vi "参数设置对画框.vi"(8 "时间等比采样":u16=10, 9 "单次采样量":u16=500, 10 "采样方式":enum16{"单采", "双重"}(ring), 11 "留样模式":T1(ring)=enum."外控留样") -> ()   [LabVIEW 2016, in "德润DR803L超标留样.lvlib"]
uses:
  <vilib>/Utility/config.llb/NI_LVConfig.lvlib
panel:
  in  "关闭":bool
  in  "打开串口":bool
  in  "释放串口":bool
  in  "超标浓度配置":bool
  # "只在停止时切换有效"
  # "只在待机时切换有效"
  # "默认：500ml（5-1000）ml （只在停止时写有效）"
  # "默认：10min（2-9999）min （只在停止时写有效）"
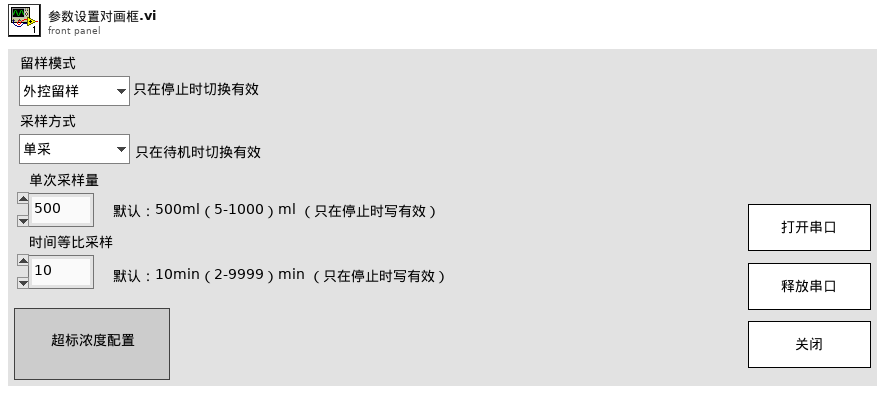
[diagram p1: front panel]
types:
  T1 = enum16{"无", "定时留样", "时间等比例", "超标留样", "同步留样", "外控留样"}
  T2 = enum16{"open", "read", "write", "write single", "close"}
  T3 = cluster{"氨氮超标浓度":dbl, "总磷超标浓度":dbl, "总氮超标浓度":dbl, "CODMn超标浓度":dbl, "CODCr超标浓度":dbl, "PH超标浓度":dbl, "DO超标浓度":dbl, "SPCOND超标浓度":dbl, "浊度超标浓度":dbl, "叶绿素a超标浓度":dbl, "蓝绿藻超标浓度":dbl, "藻密度超标浓度":dbl, "ORP超标浓度":dbl, "COD超标浓度":dbl}
  T4 = typedef "NI_LVConfig.lvlib/Config Data RefNum.ctl" = refnum<k1>
  T5 = cluster{"确定":bool, "氨氮超标浓度":dbl, "总磷超标浓度":dbl, "总氮超标浓度":dbl, "CODMn超标浓度":dbl, "CODCr超标浓度":dbl, "PH超标浓度":dbl, "DO超标浓度":dbl, "SPCOND超标浓度":dbl, "浊度超标浓度":dbl, "叶绿素a超标浓度":dbl, "蓝绿藻超标浓度":dbl, "藻密度超标浓度":dbl, "ORP超标浓度":dbl, "COD超标浓度":dbl}
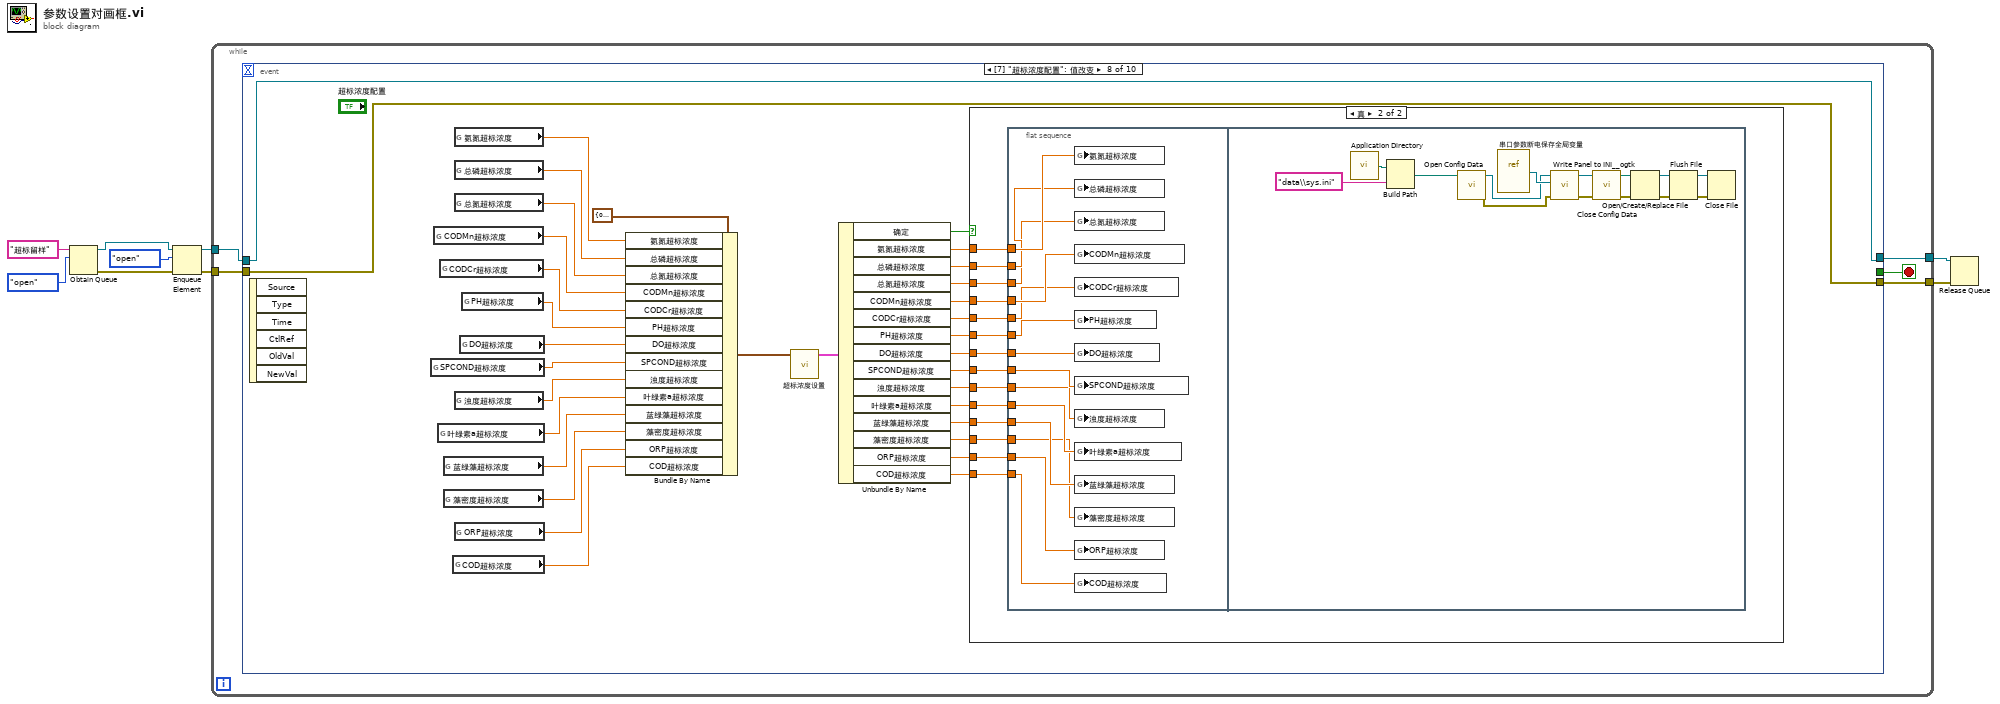
[diagram p0: block diagram]
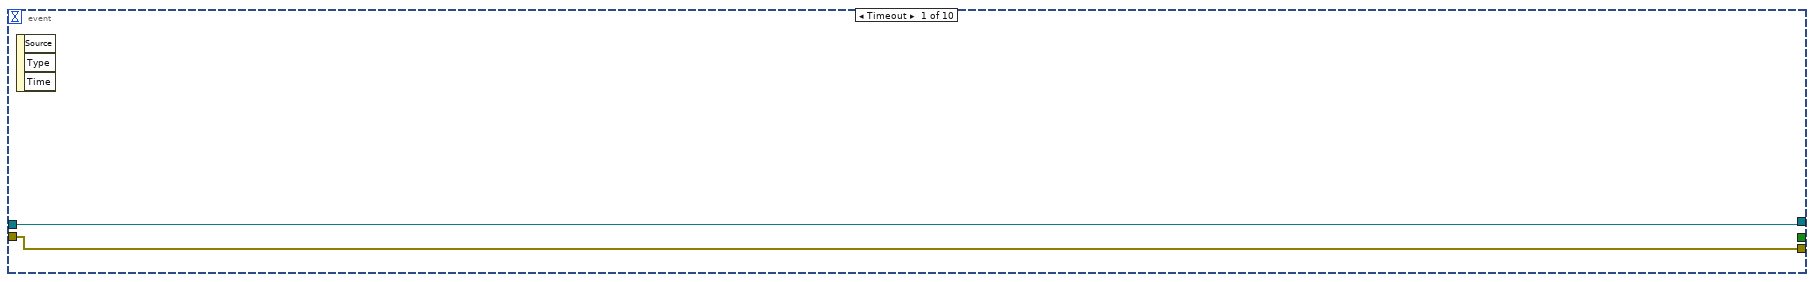
[diagram p2: hidden frame]
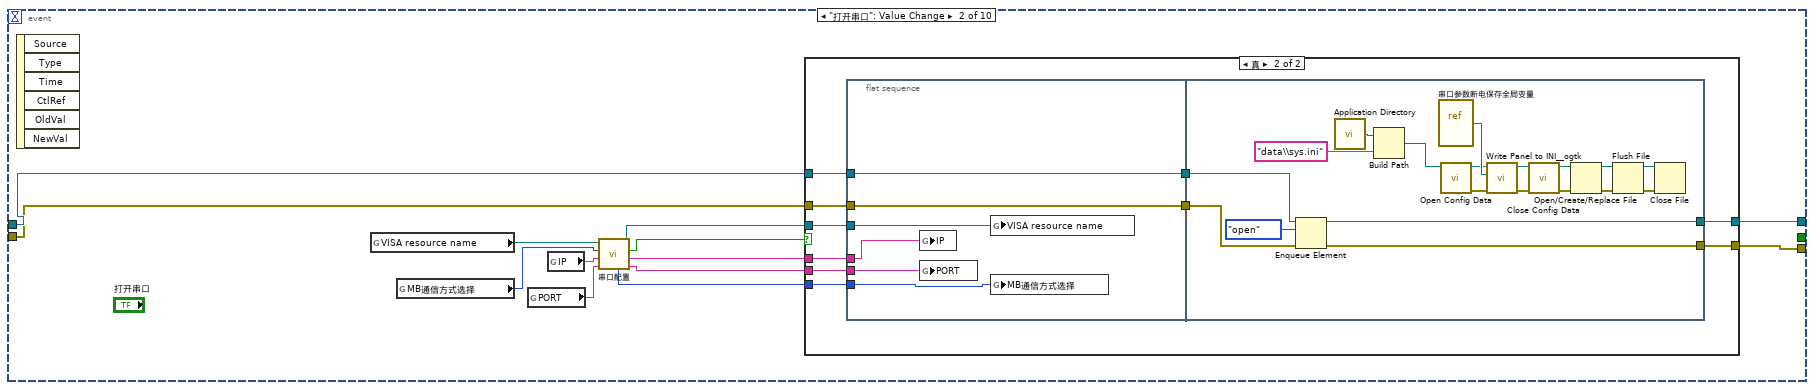
[diagram p3: hidden frame]
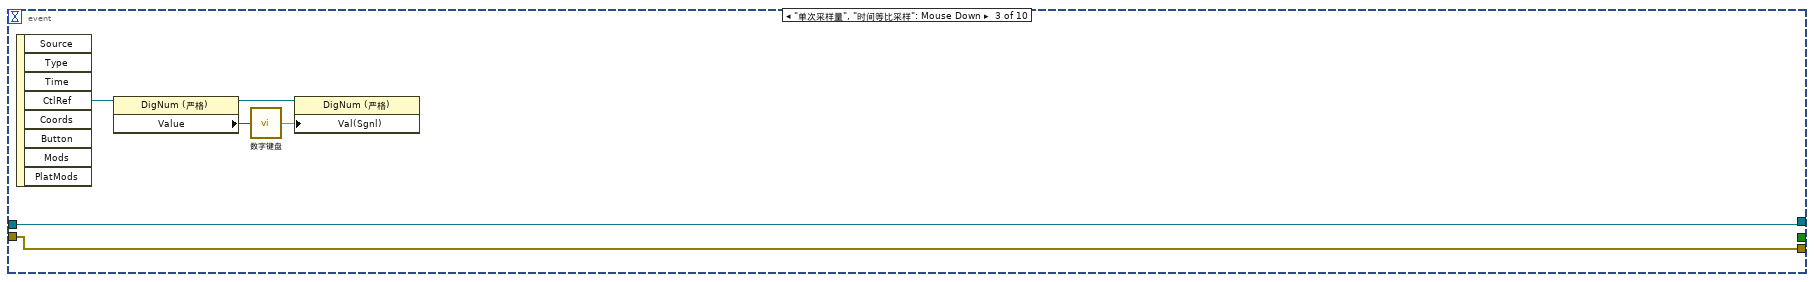
[diagram p5: hidden frame]
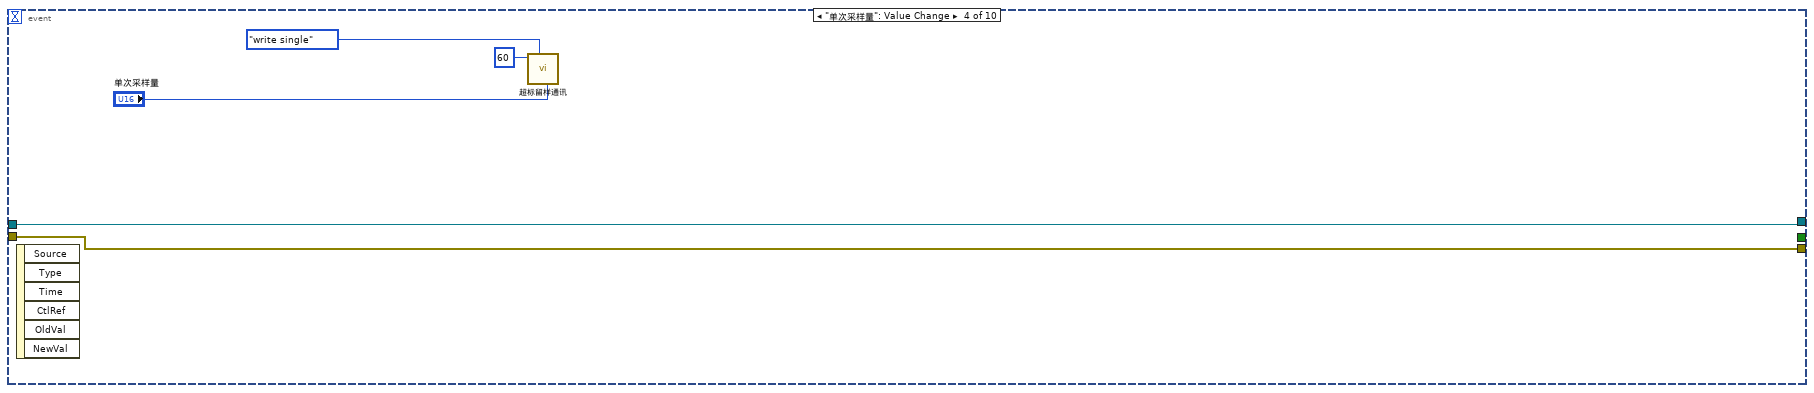
[diagram p6: hidden frame]
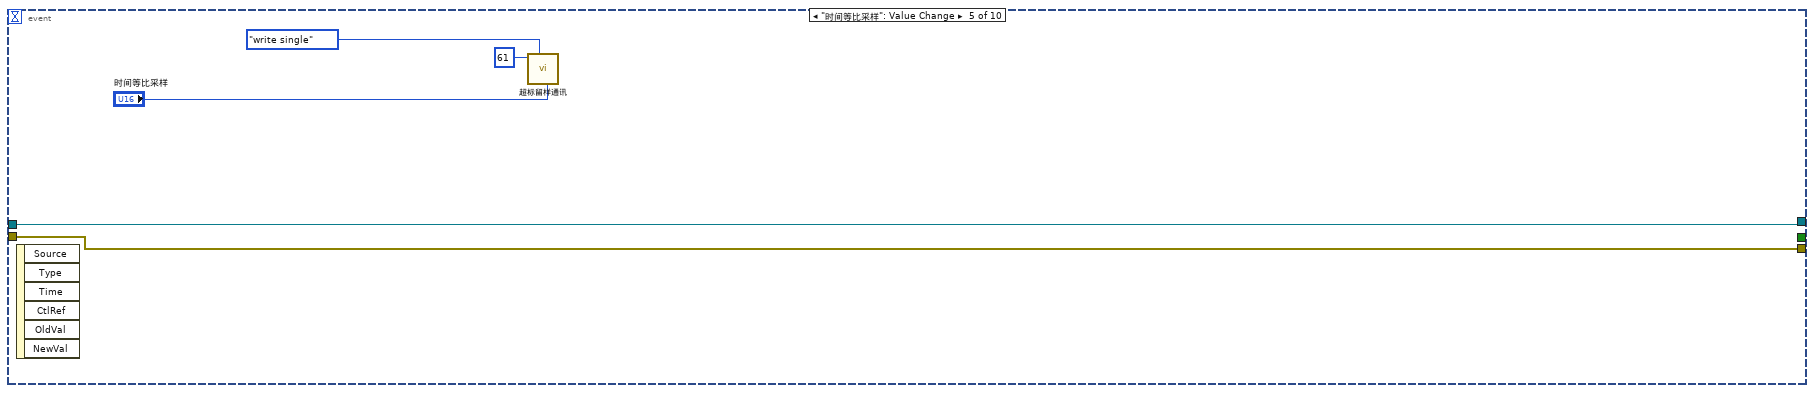
[diagram p7: hidden frame]
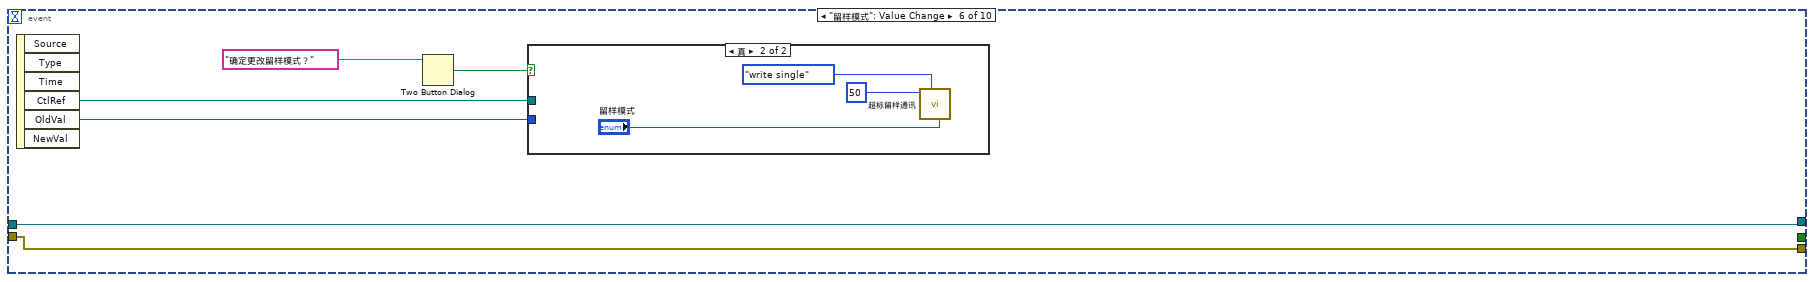
[diagram p8: hidden frame]
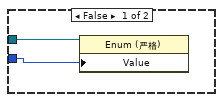
[diagram p9: hidden frame]
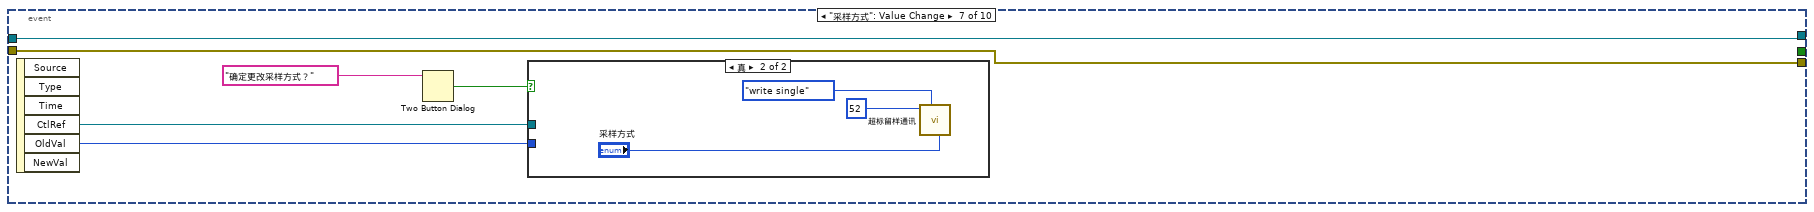
[diagram p10: hidden frame]
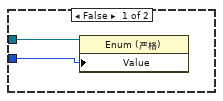
[diagram p11: hidden frame]
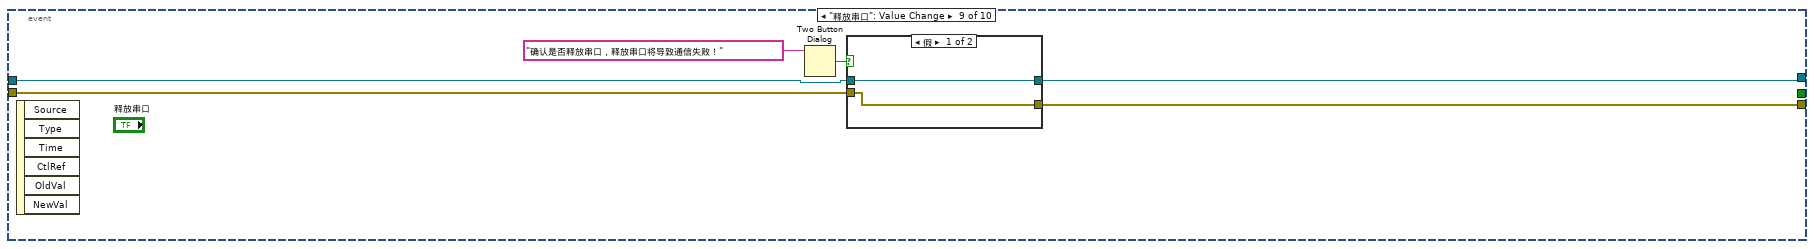
[diagram p13: hidden frame]
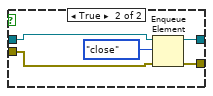
[diagram p14: hidden frame]
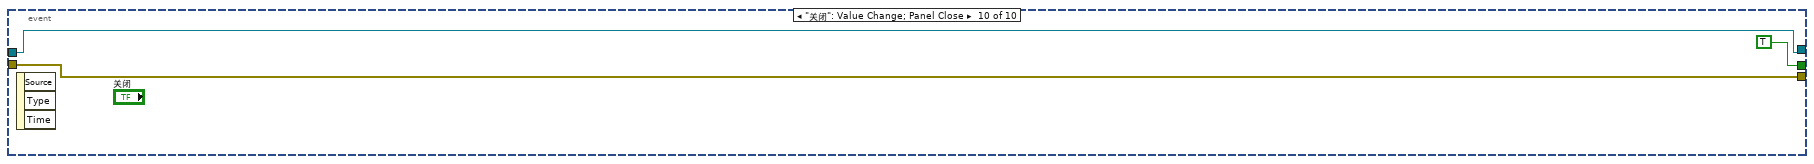
[diagram p15: hidden frame]
diagram:
  n1 = Obtain Queue(name (unnamed)="超标留样" ("名称（未命名）"), element data type=enum16{"open", "read", "write", "close"}."open") -> (queue out=w7:refnum<queue>, error out=w6:errorcluster)  [unwired: 3 in, 1 out]
  n2 = Enqueue Element(queue=w7, element=enum16{"open", "read", "write", "close"}."open", error in (no error)=w6) -> (queue out=w4:refnum<queue>, error out=w3:errorcluster)  [unwired: 1 in, 1 out]
  n3 = while {
    tunnel: w4 -> [w14]
    tunnel: w3 -> [w13]
    tunnel: [w12] -> w2
    tunnel: [w11] -> w1
    stop <- w10 stop-if-true
    n4 = event shown="[7] \"超标浓度配置\": 值改变" {
      selector: _ -> [_ _ _ _ _ _ _ _ _ _]
      dyn-events: _ -> [_ _ _ _ _ _ _ _ _ _]
      timeout: _ -> [_ _ _ _ _ _ _ _ _ _]
      tunnel: w14 -> [w16 w20 w68 w74 w79 w84 w95 w126 w184 w195]
      tunnel: w13 -> [w15 w19 w67 w73 w78 w83 w94 w125 w183 w194]
      tunnel: [w16 w18 w68 w74 w79 w84 w95 w126 w182 w195] -> w12
      tunnel: [w15 w17 w67 w73 w78 w83 w94 w125 w181 w194] -> w11
      tunnel: [_ _ _ _ _ _ _ _ _ TRUE] -> w10
      event Timeout {
        n5 = event-data() -> ()  [unwired: 1 in, 3 out]
      }
      event "打开串口": Value Change {
        n6 = event-data() -> ()  [unwired: 1 in, 6 out]
        n7 = global read "串口参数断电保存全局变量.vi" "VISA resource name"() -> (w22:refnum<visa-resource-name>)
        n8 = global read "串口参数断电保存全局变量.vi" "MB通信方式选择"() -> (w21:enum16{"串口", "TCP"})
        n9 = global read "串口参数断电保存全局变量.vi" "PORT"() -> (w24:string)
        n10 = global read "串口参数断电保存全局变量.vi" "IP"() -> (w23:string)
        n11 = call "串口配置.vi"("PORT"=w24, "IP"=w23, "MB通信方式选择"=w21, "请选择串口:"=w22) -> ("PORT 2"=w28:string, "IP 2"=w27:string, "确认 2"=w25:bool, "VISA资源名称 2"=w26:refnum<visa-resource-name>, "MB通信方式选择 2"=w29:enum16{"串口", "TCP"})  [unwired: 3 in]
        n12 = case shown="真" w25 {
          tunnel: w26 -> [_ w41]
          tunnel: w27 -> [_ w40]
          tunnel: w28 -> [_ w39]
          tunnel: w29 -> [_ w38]
          tunnel: w20 -> [w31 w37]
          tunnel: w19 -> [w30 w35]
          tunnel: [w31 w33] -> w18
          tunnel: [w30 w32] -> w17
          frame False {
          }
          frame True {
            n13 = flat-sequence {
              tunnel: w41 -> [w47]
              tunnel: w40 -> [w46]
              tunnel: w39 -> [w45]
              tunnel: w38 -> [w44]
              tunnel: w37 -> [w43]
              tunnel: [w43] -> w36
              tunnel: w35 -> [w42]
              tunnel: [w42] -> w34
              tunnel: w36 -> [w51]
              tunnel: w34 -> [w50]
              tunnel: [w49] -> w33
              tunnel: [w48] -> w32
              frame #0 {
                n14 = global write "串口参数断电保存全局变量.vi" "IP"(w46) -> ()
                n15 = global write "串口参数断电保存全局变量.vi" "PORT"(w45) -> ()
                n16 = global write "串口参数断电保存全局变量.vi" "VISA resource name"(w47) -> ()
                n17 = global write "串口参数断电保存全局变量.vi" "MB通信方式选择"(w44) -> ()
              }
              frame #1 {
                n18 = Enqueue Element(queue=w51, element=enum16{"open", "read", "write", "close"}."open" ("元素"), error in (no error)=w50) -> (queue out=w49:refnum<queue>, error out=w48:errorcluster)  [unwired: 1 in, 1 out]
                n19 = call <vilib>:"Application Directory.vi"() -> ("Application Directory"=w54:path)
                n20 = Build Path(base path=w54, name or relative path="data\\sys.ini" ("名称或相对路径")) -> (appended path=w55:path)
                n21 = vi-ref "串口参数断电保存全局变量.vi"() -> (w57:refnum<vi>)
                n22 = call <vilib>:"Open Config Data.vi"("configuration file path"=w55) -> ("error out"=w59:errorcluster, "refnum"=w56:T4)  [unwired: 8 in, 1 out]
                n23 = call <userlib>:"Write Panel to INI__ogtk.vi"("error in (no error)"=w59, "VI ref"=w57, "refnum"=w56) -> ("error out"=w60:errorcluster, "refnum out"=w58:T4)  [unwired: 7 in]
                n24 = call <vilib>:"Close Config Data.vi"("error in (no error)"=w60, "refnum"=w58) -> ("error out"=w65:errorcluster, "file path"=w66:path)  [unwired: 8 in]
                n25 = Open/Create/Replace File(file path (use dialog)=w66, error in=w65) -> (refnum out=w62:refnum<file>, error out=w61:errorcluster)  [unwired: 4 in, 1 out]
                n26 = Flush File(refnum=w62, error in=w61) -> (refnum out=w63:refnum<file>, error out=w64:errorcluster)
                n27 = Close File(refnum=w63, error in=w64) -> ()  [unwired: 2 out]
              }
            }
          }
        }
      }
      event "单次采样量", "时间等比采样": Mouse Down {
        n28 = event-data() -> ("CtlRef"=w69:refnum<vi>)  [unwired: 1 in, 7 out]
        n29 = property class="DigNum (严格)"(reference=w69) -> (reference out=w72:refnum<vi>, "Value"=w71:u16)  [unwired: 1 in, 1 out]
        n30 = call "数字键盘.vi"("OldNumber"=w71) -> ("NewNumber"=w70:sgl)
        n31 = property class="DigNum (严格)"(reference=w72, "Val(Sgnl)"=w70) -> ()  [unwired: 1 in, 2 out]
      }
      event "单次采样量": Value Change {
        n32 = event-data() -> ()  [unwired: 1 in, 6 out]
        n33 = call "超标留样通讯.vi"("value"="单次采样量", "STEP"=T2."write single", "starting address"=60 ("索引")) -> ()  [unwired: 6 in, 3 out]
      }
      event "时间等比采样": Value Change {
        n34 = event-data() -> ()  [unwired: 1 in, 6 out]
        n35 = call "超标留样通讯.vi"("value"="时间等比采样", "STEP"=T2."write single", "starting address"=61 ("索引")) -> ()  [unwired: 6 in, 3 out]
      }
      event "留样模式": Value Change {
        n36 = event-data() -> ("CtlRef"=w86:refnum<vi>, "OldVal"=w85:T1)  [unwired: 1 in, 4 out]
        n37 = Two Button Dialog(message="确定更改留样模式？" ("消息")) -> (T button?=w87:bool)  [unwired: 2 in]
        n38 = case shown="真" w87 {
          tunnel: w85 -> [w89 _]
          tunnel: w86 -> [w90 _]
          frame False {
            n39 = property class="Enum (严格)"(reference=w90, "Value"=w89) -> ()  [unwired: 1 in, 2 out]
          }
          frame True {
            n40 = call "超标留样通讯.vi"("value"="留样模式", "STEP"=T2."write single", "starting address"=50 ("索引")) -> ()  [unwired: 6 in, 3 out]
          }
        }
      }
      event "采样方式": Value Change {
        n41 = event-data() -> ("CtlRef"=w97:refnum<vi>, "OldVal"=w96:enum16{"单采", "双重"})  [unwired: 1 in, 4 out]
        n42 = Two Button Dialog(message="确定更改采样方式？" ("消息")) -> (T button?=w98:bool)  [unwired: 2 in]
        n43 = case shown="真" w98 {
          tunnel: w97 -> [w101 _]
          tunnel: w96 -> [w100 _]
          frame False {
            n44 = property class="Enum (严格)"(reference=w101, "Value"=w100) -> ()  [unwired: 1 in, 2 out]
          }
          frame True {
            n45 = call "超标留样通讯.vi"("value"="采样方式", "STEP"=T2."write single", "starting address"=52 ("索引")) -> ()  [unwired: 6 in, 3 out]
          }
        }
      }
      event "超标浓度配置": Value Change {
        n46 = event-data() -> ()  [unwired: 1 in, 6 out]
        n47 = global read "串口参数断电保存全局变量.vi" "SPCOND超标浓度"() -> (w121:dbl)
        n48 = global read "串口参数断电保存全局变量.vi" "CODMn超标浓度"() -> (w137:dbl)
        n49 = global read "串口参数断电保存全局变量.vi" "叶绿素a超标浓度"() -> (w119:dbl)
        n50 = global read "串口参数断电保存全局变量.vi" "CODCr超标浓度"() -> (w136:dbl)
        n51 = global read "串口参数断电保存全局变量.vi" "蓝绿藻超标浓度"() -> (w118:dbl)
        n52 = global read "串口参数断电保存全局变量.vi" "藻密度超标浓度"() -> (w117:dbl)
        n53 = global read "串口参数断电保存全局变量.vi" "COD超标浓度"() -> (w115:dbl)
        n54 = global read "串口参数断电保存全局变量.vi" "氨氮超标浓度"() -> (w135:dbl)
        n55 = global read "串口参数断电保存全局变量.vi" "总磷超标浓度"() -> (w134:dbl)
        n56 = global read "串口参数断电保存全局变量.vi" "总氮超标浓度"() -> (w138:dbl)
        n57 = global read "串口参数断电保存全局变量.vi" "浊度超标浓度"() -> (w120:dbl)
        n58 = global read "串口参数断电保存全局变量.vi" "ORP超标浓度"() -> (w116:dbl)
        n59 = global read "串口参数断电保存全局变量.vi" "DO超标浓度"() -> (w122:dbl)
        n60 = global read "串口参数断电保存全局变量.vi" "PH超标浓度"() -> (w123:dbl)
        n61 = Bundle By Name(cluster=T3 {"氨氮超标浓度"=0.0, "总磷超标浓度"=0.0, "总氮超标浓度"=0.0, "CODMn超标浓度"=0.0, "CODCr超标浓度"=0.0, "PH超标浓度"=0.0, "DO超标浓度"=0.0, "SPCOND超标浓度"=0.0, "浊度超标浓度"=0.0, "叶绿素a超标浓度"=0.0, "蓝绿藻超标浓度"=0.0, "藻密度超标浓度"=0.0, "ORP超标浓度"=0.0, "COD超标浓度"=0.0} ("输入"), "氨氮超标浓度"=w135, "总磷超标浓度"=w134, "总氮超标浓度"=w138, "CODMn超标浓度"=w137, "CODCr超标浓度"=w136, "PH超标浓度"=w123, "DO超标浓度"=w122, "SPCOND超标浓度"=w121, "浊度超标浓度"=w120, "叶绿素a超标浓度"=w119, "蓝绿藻超标浓度"=w118, "藻密度超标浓度"=w117, "ORP超标浓度"=w116, "COD超标浓度"=w115) -> (w105:T3)
        n62 = call "超标浓度设置.vi"("输入"=w105) -> ("输出"=w133:T5)  [unwired: 10 in]
        n63 = Unbundle By Name(w133) -> ("确定"=w132:bool, "氨氮超标浓度"=w131:dbl, "总磷超标浓度"=w130:dbl, "总氮超标浓度"=w129:dbl, "CODMn超标浓度"=w128:dbl, "CODCr超标浓度"=w127:dbl, "PH超标浓度"=w114:dbl, "DO超标浓度"=w113:dbl, "SPCOND超标浓度"=w112:dbl, "浊度超标浓度"=w111:dbl, "叶绿素a超标浓度"=w110:dbl, "蓝绿藻超标浓度"=w109:dbl, "藻密度超标浓度"=w108:dbl, "ORP超标浓度"=w107:dbl, "COD超标浓度"=w106:dbl)
        n64 = case shown="真" w132 {
          tunnel: w131 -> [_ w152]
          tunnel: w130 -> [_ w151]
          tunnel: w129 -> [_ w150]
          tunnel: w128 -> [_ w149]
          tunnel: w127 -> [_ w148]
          tunnel: w114 -> [_ w147]
          tunnel: w113 -> [_ w146]
          tunnel: w112 -> [_ w145]
          tunnel: w111 -> [_ w144]
          tunnel: w110 -> [_ w143]
          tunnel: w109 -> [_ w142]
          tunnel: w108 -> [_ w141]
          tunnel: w107 -> [_ w140]
          tunnel: w106 -> [_ w139]
          frame False {
          }
          frame True {
            n65 = flat-sequence {
              tunnel: w152 -> [w166]
              tunnel: w151 -> [w165]
              tunnel: w150 -> [w164]
              tunnel: w149 -> [w163]
              tunnel: w148 -> [w162]
              tunnel: w147 -> [w161]
              tunnel: w146 -> [w160]
              tunnel: w145 -> [w159]
              tunnel: w144 -> [w158]
              tunnel: w143 -> [w157]
              tunnel: w142 -> [w156]
              tunnel: w141 -> [w155]
              tunnel: w140 -> [w154]
              tunnel: w139 -> [w153]
              frame #0 {
                n66 = global write "串口参数断电保存全局变量.vi" "氨氮超标浓度"(w166) -> ()
                n67 = global write "串口参数断电保存全局变量.vi" "总磷超标浓度"(w165) -> ()
                n68 = global write "串口参数断电保存全局变量.vi" "总氮超标浓度"(w164) -> ()
                n69 = global write "串口参数断电保存全局变量.vi" "CODMn超标浓度"(w163) -> ()
                n70 = global write "串口参数断电保存全局变量.vi" "CODCr超标浓度"(w162) -> ()
                n71 = global write "串口参数断电保存全局变量.vi" "PH超标浓度"(w161) -> ()
                n72 = global write "串口参数断电保存全局变量.vi" "DO超标浓度"(w160) -> ()
                n73 = global write "串口参数断电保存全局变量.vi" "SPCOND超标浓度"(w159) -> ()
                n74 = global write "串口参数断电保存全局变量.vi" "浊度超标浓度"(w158) -> ()
                n75 = global write "串口参数断电保存全局变量.vi" "叶绿素a超标浓度"(w157) -> ()
                n76 = global write "串口参数断电保存全局变量.vi" "蓝绿藻超标浓度"(w156) -> ()
                n77 = global write "串口参数断电保存全局变量.vi" "藻密度超标浓度"(w155) -> ()
                n78 = global write "串口参数断电保存全局变量.vi" "ORP超标浓度"(w154) -> ()
                n79 = global write "串口参数断电保存全局变量.vi" "COD超标浓度"(w153) -> ()
              }
              frame #1 {
                n80 = call <vilib>:"Application Directory.vi"() -> ("Application Directory"=w168:path)
                n81 = Build Path(base path=w168, name or relative path="data\\sys.ini" ("名称或相对路径")) -> (appended path=w169:path)
                n82 = call <vilib>:"Open Config Data.vi"("configuration file path"=w169) -> ("error out"=w173:errorcluster, "refnum"=w170:T4)  [unwired: 8 in, 1 out]
                n83 = vi-ref "串口参数断电保存全局变量.vi"() -> (w171:refnum<vi>)
                n84 = call <userlib>:"Write Panel to INI__ogtk.vi"("error in (no error)"=w173, "VI ref"=w171, "refnum"=w170) -> ("error out"=w174:errorcluster, "refnum out"=w172:T4)  [unwired: 7 in]
                n85 = call <vilib>:"Close Config Data.vi"("error in (no error)"=w174, "refnum"=w172) -> ("error out"=w179:errorcluster, "file path"=w180:path)  [unwired: 8 in]
                n86 = Open/Create/Replace File(file path (use dialog)=w180, error in=w179) -> (refnum out=w176:refnum<file>, error out=w175:errorcluster)  [unwired: 4 in, 1 out]
                n87 = Flush File(refnum=w176, error in=w175) -> (refnum out=w177:refnum<file>, error out=w178:errorcluster)
                n88 = Close File(refnum=w177, error in=w178) -> ()  [unwired: 2 out]
              }
            }
          }
        }
      }
      event "释放串口": Value Change {
        n89 = event-data() -> ()  [unwired: 1 in, 6 out]
        n90 = Two Button Dialog(message="确认是否释放串口，释放串口将导致通信失败！" ("消息")) -> (T button?=w185:bool)  [unwired: 2 in]
        n91 = case shown="假" w185 {
          tunnel: w184 -> [w188 w192]
          tunnel: w183 -> [w187 w191]
          tunnel: [w188 w190] -> w182
          tunnel: [w187 w189] -> w181
          frame False {
          }
          frame True {
            n92 = Enqueue Element(queue=w192, element=enum16{"open", "read", "write", "close"}."close" ("元素"), error in (no error)=w191) -> (queue out=w190:refnum<queue>, error out=w189:errorcluster)  [unwired: 1 in, 1 out]
          }
        }
      }
      event "关闭": Value Change; Panel Close {
        n93 = event-data() -> ()  [unwired: 1 in, 3 out]
      }
    }
  }
  n94 = Release Queue(queue=w2, error in (no error)=w1) -> ()  [unwired: 1 in, 3 out]
